vi "Get Capabilities.vi"(0 "reference in":refnum<class "Simulated-PowerModule.lvclass">, 11 "Error In":errorcluster) -> (4 "reference out":refnum<class "Simulated-PowerModule.lvclass">, 6 "modes":string[](array[string]), 8 "ranges":string[](array[string]), 15 "Error Out":errorcluster)   [LabVIEW 2023, in "Simulated-PowerModule.lvlib" / "Simulated-PowerModule.lvclass"]
uses:
  Simulated-PowerModule.lvclass
  Mode.ctl
  Range.ctl
  Simulated-PowerModule.lvclass/Simulated-PowerModule.ctl
panel:
  in  "RANGE":T1 items=["0,1500 V / -240,240 A"]
  in  "MODE":T2 items=["CONSTANT CURRENT & VOLTAGE"]
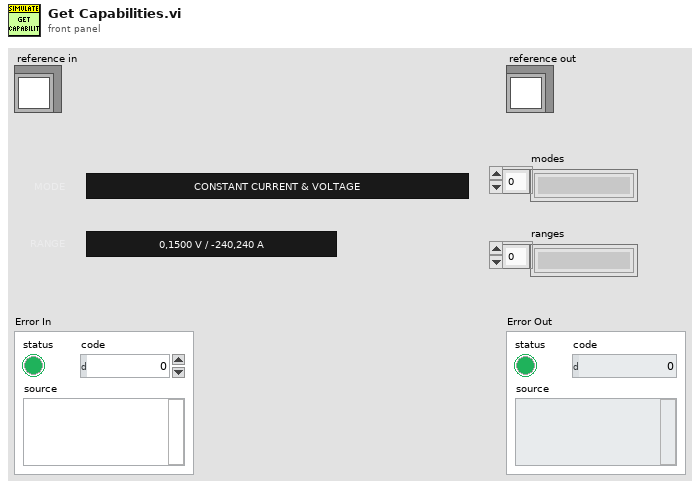
[diagram p1: front panel]
types:
  T1 = typedef "Simulated-PowerModule.lvlib/Simulated-PowerModule.lvclass/Range.ctl" = u16
  T2 = typedef "Simulated-PowerModule.lvlib/Simulated-PowerModule.lvclass/Mode.ctl" = u16
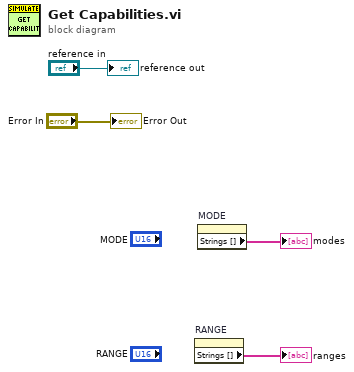
[diagram p0: block diagram]
diagram:
  n1 = property on="RANGE" class="Ring (strict)"() -> ("Strings []"=→"ranges":string[])  [unwired: 2 in, 2 out]
  n2 = property on="MODE" class="Ring (strict)"() -> ("Strings []"=→"modes":string[])  [unwired: 2 in, 2 out]
  "Error Out" <- "Error In"
  "reference out" <- "reference in"
